vi "Block FFT.vi"(2 "window coefficients":dbl[](array[numeric]) format="%.2f", 3 "X":dbl[](array[numeric]) format="%.2f") -> (0 "Last Spectrum":cluster{"x[i]":dbl[], "y[i]":dbl[]} {"y[i]" format="%.2f"; "x[i]" format="%.2f"}, 1 "Block FFT Spectrum":dbl[][](array[numeric]) format="%.2f")   [LabVIEW 2017]
doc: "Computes the signal energy distribution in the joint time-frequency domain using the Short-Time Fourier Transform (STFT). This VI performs a sliding FFT."
uses:
  <vilib>/Analysis/1siggen.llb/Ramp Pattern by Samples.vi
  <vilib>/Analysis/NI_AALPro.lvlib
  <vilib>/Analysis/NI_AALBase.lvlib
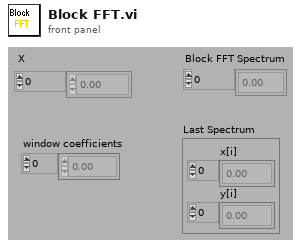
[diagram p1: front panel]
types:
  T1 = cluster{"Power Spectrum (V^2 rms)":dbl[], "Ramp Pattern":dbl[]}
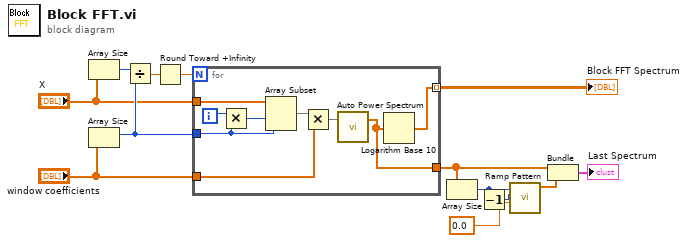
[diagram p0: block diagram]
diagram:
  n1 = Array Size(array="X") -> (size(s)=w13:i32)
  n2 = Array Size(array="window coefficients") -> (size(s)=w10:i32)
  n3 = Divide(x=w13, y=w10) -> (x/y=w12:dbl)
  n4 = Round Toward +Infinity(x=w12) -> (ceil(x): smallest int >= x=w11:dbl)
  n5 = for {
    N: w11 -> [_]
    tunnel: w10 -> [w17]
    tunnel: "X" -> [w21]
    tunnel: "window coefficients" -> [w19]
    tunnel: [w15] -> w1 mode=indexing
    tunnel: [w14] -> w3
    i -> [w16]
    n6 = Multiply(x=w16, y=w17) -> (x*y=w22:i32)
    n7 = Array Subset(array=w21, index=w22, length=w17) -> (w20:dbl[])
    n8 = Multiply(x=w20, y=w19) -> (x*y=w18:dbl[])
    n9 = call <vilib>:"Auto Power Spectrum.vi"("Signal (V)"=w18) -> ("Power Spectrum (V^2 rms)"=w14:dbl[])  [unwired: 1 in, 1 out]
    n10 = Logarithm Base 10(1:w14) -> (0:w15:dbl[])
  }
  "Block FFT Spectrum" <- w1
  n11 = Array Size(array=w3) -> (size(s)=w7:i32)
  n12 = Decrement(x=w7) -> (x-1=w6:i32)
  n13 = call-poly <vilib>:"Ramp Pattern.vi"("start"=0.0, "end"=w6, "samples"=w7) -> ("Ramp Pattern"=w2:dbl[])  [unwired: 7 in, 1 out]
  n14 = Bundle("Power Spectrum (V^2 rms)"=w3, "Ramp Pattern"=w2) -> (→"Last Spectrum":T1)  [unwired: 1 in]
